vi "Cluster to String.vi"(1 "Correlator Initial Data":T1={"Max Exposition Time (ms)"=1, "Channel1 Threshold Voltage (mV)"=1, "Channel1 Pulse Front"="", "Channel2 Threshold Voltage (mV)"=1, "Channel2 Pulse Front"="", "Channel3 Threshold Voltage (mV)"=1, "Channel3 Pulse Front "="", "Channel4 Threshold Voltage (mV)"=1, "Channel4 Pulse Front "="", "Single Count Enable"={"Channel1"=FALSE, "Channel2"=FALSE, "Channel3"=FALSE, "Channel4"=FALSE}, "Single Count Max"=1, "Sum Count Enable"={"Channel1"=FALSE, "Channel2"=FALSE, "Channel3"=FALSE, "Channel4"=FALSE}, "Sum Count Max"=1, "Start-Stop1 Multyplex"={"Stop Channel"="", "Start Channel"=""}, "Stop Delay 1 (ns)"=1, "Window Length 1 (ns)"=4, "Window Offset 1 (ns) "=4, "Conditional Correlation 1"="", "Histogram Bin 1"="", "Histogram Start 1 (ns) "=4, "Start-Stop2 Multyplex "={"Stop Channel"="", "Start Channel"=""}, "Stop Delay 2 (ns)"=1, "Window Length 2 (ns) "=4, "Window Offset 2 (ns) "=4, "Conditional Correlation 2"="", "Histogram Bin 2"="", "Histogram Start 2 (ns)  "=4, "Start-Stop3 Multyplex"={"Stop Channel"="", "Start Channel"=""}, "Stop Delay 3 (ns)"=1, "Window Length 3 (ns) "=4, "Window Offset 3 (ns) "=4, "Conditional Correlation 3"="", "Histogram Bin 3"="", "Histogram Start 3 (ns) "=4, "Start-Stop4 Multyplex"={"Stop Channel"="", "Start Channel"=""}, "Stop Delay 4 (ns)"=1, "Window Length 4 (ns)  "=4, "Window Offset 4 (ns) "=4, "Conditional Correlation 4"="", "Histogram Bin 4"="", "Histogram Start 4 (ns)  "=4, "Coincidence Count Enable"={"Start-Stop1"=FALSE, "Start-Stop2"=FALSE, "Start-Stop3"=FALSE, "Start-Stop4"=FALSE}, "Coincidence Count Max"=1, "Coincidence Sum Enable 2"={"Start-Stop1"=FALSE, "Start-Stop2"=FALSE, "Start-Stop3"=FALSE, "Start-Stop4"=FALSE}, "Coincidence Sum Max"=1, "Output Channel Enable"={"Channel1"=FALSE, "Channel2"=FALSE, "Channel3"=FALSE, "Channel4"=FALSE}, "Output Channel Inversion"={"Channel1"=FALSE, "Channel2"=FALSE, "Channel3"=FALSE, "Channel4"=FALSE, "Output"=FALSE}} {"Coincidence Sum Max" min=1 max=16777215 step=1 format="%.7e"; "Coincidence Count Max" min=1 max=16777215 step=1 format="%.7e"; "Histogram Start 4 (ns)" min=0 max=120000 step=2; "Window Offset 4 (ns)" min=0 max=120000 step=2; "Window Length 4 (ns)" min=4 max=60000 step=4; "Stop Delay 4 (ns)" min=0 max=1008 step=16; "Histogram Start 3 (ns)" min=0 max=120000 step=2; "Window Offset 3 (ns)" min=0 max=120000 step=2; "Window Length 3 (ns)" min=4 max=60000 step=4; "Stop Delay 3 (ns)" min=0 max=1008 step=16; "Histogram Start 2 (ns)" min=0 max=120000 step=2; "Window Offset 2 (ns)" min=0 max=120000 step=2; "Window Length 2 (ns)" min=4 max=60000 step=4; "Stop Delay 2 (ns)" min=0 max=1008 step=16; "Histogram Start 1 (ns)" min=0 max=120000 step=2; "Window Offset 1 (ns)" min=0 max=120000 step=2; "Window Length 1 (ns)" min=4 max=60000 step=4; "Stop Delay 1 (ns)" min=0 max=1008 step=16; "Sum Count Max" min=1 max=16777215 step=1 format="%.7e"; "Single Count Max" min=1 max=16777215 step=1 format="%.7e"; "Channel4 Threshold Voltage (mV)" min=0 max=5000 step=10; "Channel3 Threshold Voltage (mV)" min=0 max=5000 step=10; "Channel2 Threshold Voltage (mV)" min=0 max=5000 step=10; "Channel1 Threshold Voltage (mV)" min=0 max=5000 step=10; "Max Exposition Time (ms)" min=1 max=3600000000 step=1 format="%.9e"}) -> (0 "string":string)   [LabVIEW 2012]
panel:
  out "Input":i64[](array[numeric])
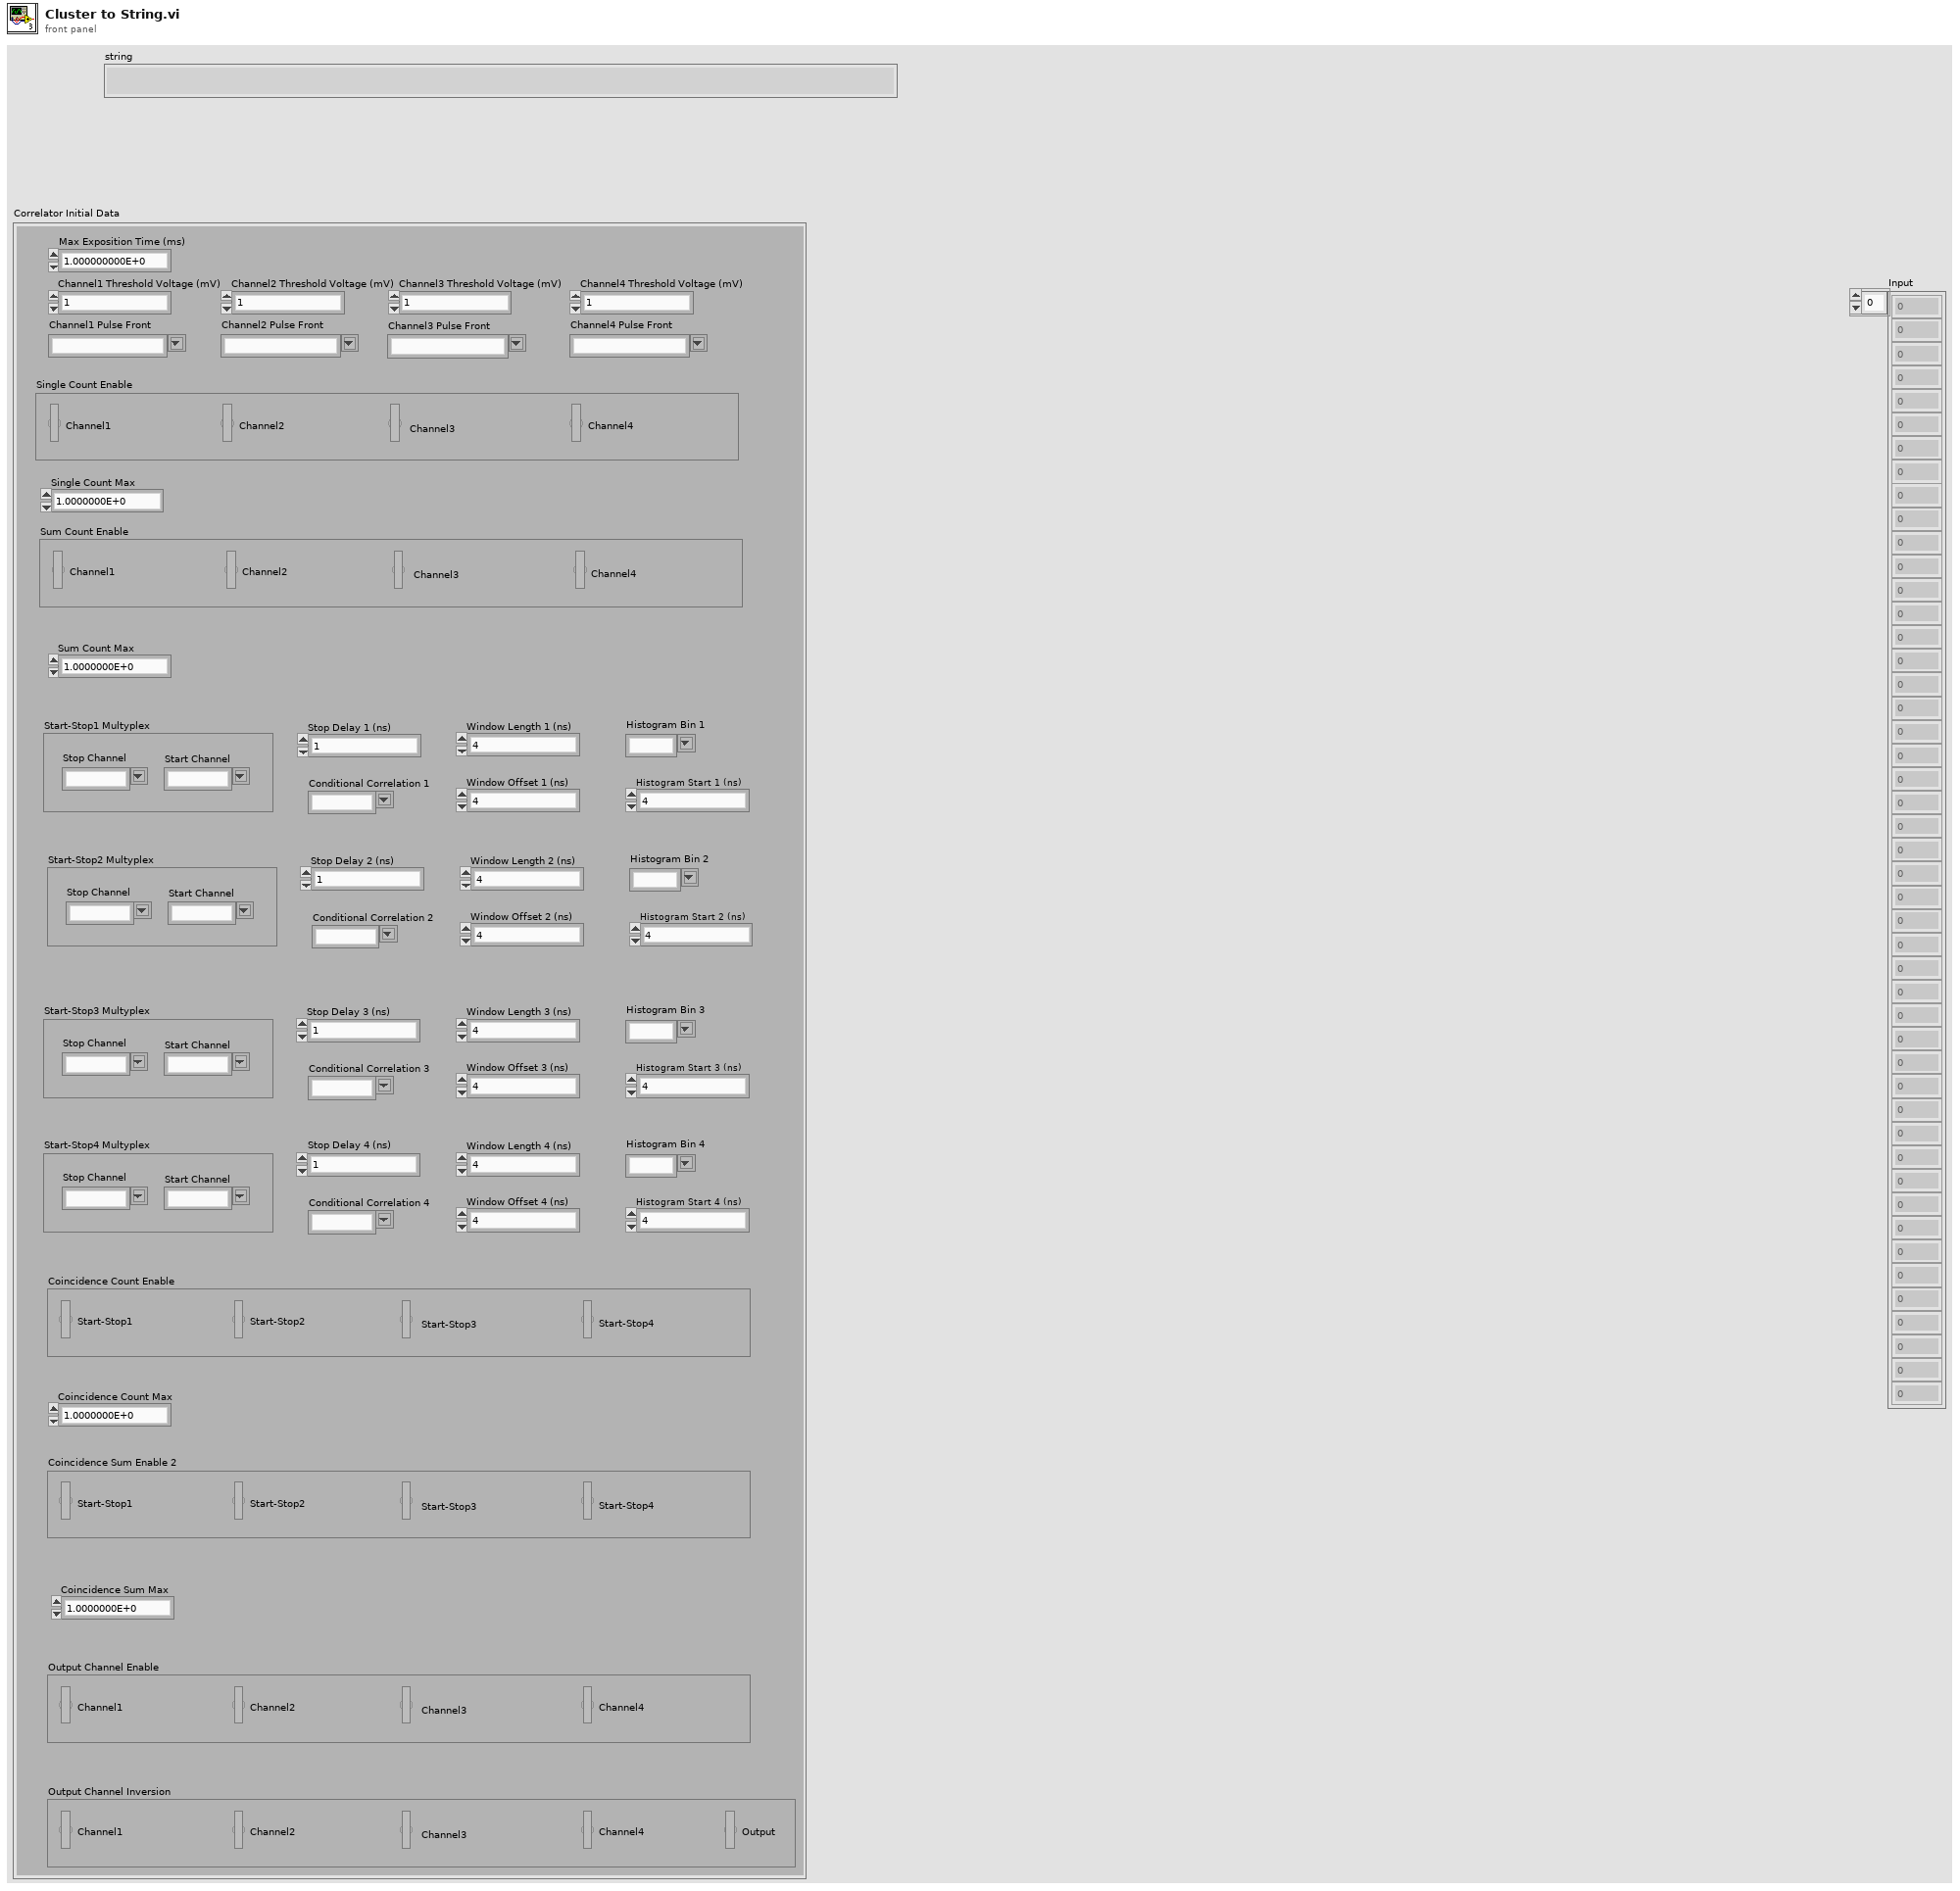
[diagram p1: front panel]
types:
  T1 = cluster{"Max Exposition Time (ms)":i64, "Channel1 Threshold Voltage (mV)":i32, "Channel1 Pulse Front":string, "Channel2 Threshold Voltage (mV)":i32, "Channel2 Pulse Front":string, "Channel3 Threshold Voltage (mV)":i32, "Channel3 Pulse Front ":string, "Channel4 Threshold Voltage (mV)":i32, "Channel4 Pulse Front ":string, "Single Count Enable":cluster{"Channel1":bool, "Channel2":bool, "Channel3":bool, "Channel4":bool}, "Single Count Max":i32, "Sum Count Enable":cluster{"Channel1":bool, "Channel2":bool, "Channel3":bool, "Channel4":bool}, "Sum Count Max":i32, "Start-Stop1 Multyplex":cluster{"Stop Channel":string, "Start Channel":string}, "Stop Delay 1 (ns)":i16, "Window Length 1 (ns)":i32, "Window Offset 1 (ns) ":i32, "Conditional Correlation 1":string, "Histogram Bin 1":string, "Histogram Start 1 (ns) ":i32, "Start-Stop2 Multyplex ":cluster{"Stop Channel":string, "Start Channel":string}, "Stop Delay 2 (ns)":i16, "Window Length 2 (ns) ":i32, "Window Offset 2 (ns) ":i32, "Conditional Correlation 2":string, "Histogram Bin 2":string, "Histogram Start 2 (ns)  ":i32, "Start-Stop3 Multyplex":cluster{"Stop Channel":string, "Start Channel":string}, "Stop Delay 3 (ns)":i16, "Window Length 3 (ns) ":i32, "Window Offset 3 (ns) ":i32, "Conditional Correlation 3":string, "Histogram Bin 3":string, "Histogram Start 3 (ns) ":i32, "Start-Stop4 Multyplex":cluster{"Stop Channel":string, "Start Channel":string}, "Stop Delay 4 (ns)":i16, "Window Length 4 (ns)  ":i32, "Window Offset 4 (ns) ":i32, "Conditional Correlation 4":string, "Histogram Bin 4":string, "Histogram Start 4 (ns)  ":i32, "Coincidence Count Enable":cluster{"Start-Stop1":bool, "Start-Stop2":bool, "Start-Stop3":bool, "Start-Stop4":bool}, "Coincidence Count Max":i32, "Coincidence Sum Enable 2":cluster{"Start-Stop1":bool, "Start-Stop2":bool, "Start-Stop3":bool, "Start-Stop4":bool}, "Coincidence Sum Max":i32, "Output Channel Enable":cluster{"Channel1":bool, "Channel2":bool, "Channel3":bool, "Channel4":bool}, "Output Channel Inversion":cluster{"Channel1":bool, "Channel2":bool, "Channel3":bool, "Channel4":bool, "Output":bool}}
  T2 = cluster{"Channel1":bool, "Channel2":bool, "Channel3":bool, "Channel4":bool}
  T3 = cluster{"Stop Channel":string, "Start Channel":string}
  T4 = cluster{"Start-Stop1":bool, "Start-Stop2":bool, "Start-Stop3":bool, "Start-Stop4":bool}
  T5 = cluster{"Channel1":bool, "Channel2":bool, "Channel3":bool, "Channel4":bool, "Output":bool}
  T6 = cluster{"Channel1 Pulse Front":string, "Channel2 Pulse Front":string, "Channel3 Pulse Front ":string, "Channel4 Pulse Front ":string, "Conditional Correlation 1":string, "Histogram Bin 1":string, "Conditional Correlation 2":string, "Histogram Bin 2":string, "Conditional Correlation 3":string, "Histogram Bin 3":string, "Conditional Correlation 4":string, "Histogram Bin 4":string}
  T7 = cluster{"Channel1 Pulse Front":u32, "Channel2 Pulse Front":u32, "Channel3 Pulse Front ":u32, "Channel4 Pulse Front ":u32, "Conditional Correlation 1":u32, "Histogram Bin 1":u32, "Conditional Correlation 2":u32, "Histogram Bin 2":u32, "Conditional Correlation 3":u32, "Histogram Bin 3":u32, "Conditional Correlation 4":u32, "Histogram Bin 4":u32}
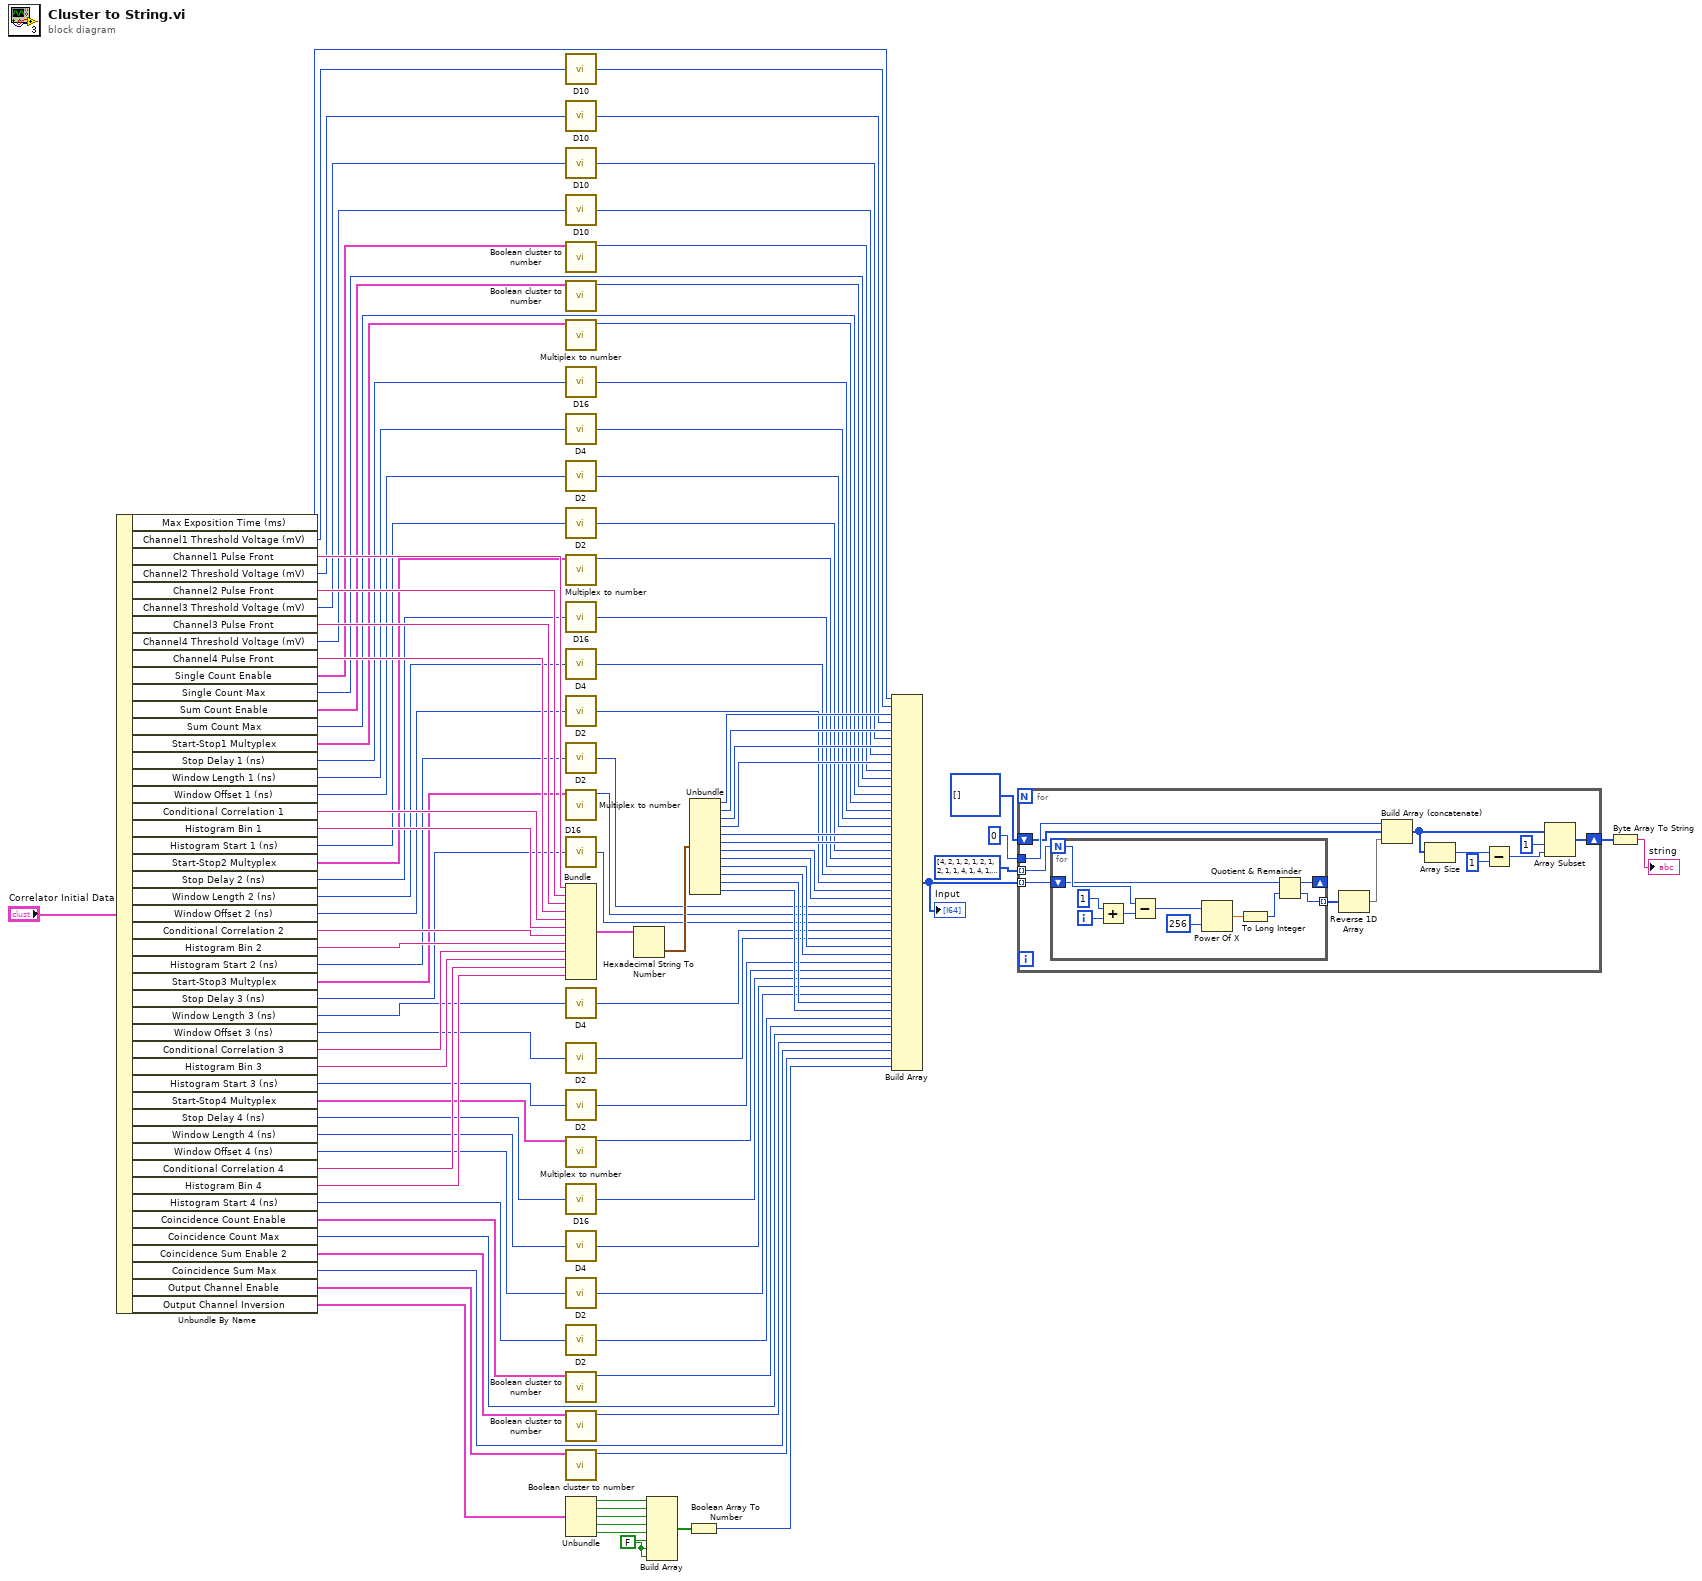
[diagram p0: block diagram]
diagram:
  w48 = FALSE ("element")
  n1 = Unbundle By Name("Correlator Initial Data") -> ("Max Exposition Time (ms)"=w76:i64, "Channel1 Threshold Voltage (mV)"=w75:i32, "Channel1 Pulse Front"=w105:string, "Channel2 Threshold Voltage (mV)"=w74:i32, "Channel2 Pulse Front"=w104:string, "Channel3 Threshold Voltage (mV)"=w73:i32, "Channel3 Pulse Front"=w103:string, "Channel4 Threshold Voltage (mV)"=w72:i32, "Channel4 Pulse Front"=w102:string, "Single Count Enable"=w42:T2, "Single Count Max"=w71:i32, "Sum Count Enable"=w41:T2, "Sum Count Max"=w70:i32, "Start-Stop1 Multyplex"=w81:T3, "Stop Delay 1 (ns)"=w69:i16, "Window Length 1 (ns)"=w68:i32, "Window Offset 1 (ns)"=w67:i32, "Conditional Correlation 1"=w101:string, "Histogram Bin 1"=w100:string, "Histogram Start 1 (ns)"=w66:i32, "Start-Stop2 Multyplex"=w79:T3, "Stop Delay 2 (ns)"=w65:i16, "Window Length 2 (ns)"=w64:i32, "Window Offset 2 (ns)"=w63:i32, "Conditional Correlation 2"=w99:string, "Histogram Bin 2"=w98:string, "Histogram Start 2 (ns)"=w62:i32, "Start-Stop3 Multyplex"=w77:T3, "Stop Delay 3 (ns)"=w61:i16, "Window Length 3 (ns)"=w60:i32, "Window Offset 3 (ns)"=w59:i32, "Conditional Correlation 3"=w97:string, "Histogram Bin 3"=w96:string, "Histogram Start 3 (ns)"=w58:i32, "Start-Stop4 Multyplex"=w82:T3, "Stop Delay 4 (ns)"=w57:i16, "Window Length 4 (ns)"=w56:i32, "Window Offset 4 (ns)"=w55:i32, "Conditional Correlation 4"=w95:string, "Histogram Bin 4"=w94:string, "Histogram Start 4 (ns)"=w54:i32, "Coincidence Count Enable"=w45:T4, "Coincidence Count Max"=w20:i32, "Coincidence Sum Enable 2"=w43:T4, "Coincidence Sum Max"=w22:i32, "Output Channel Enable"=w44:T2, "Output Channel Inversion"=w47:T5)
  n2 = call "D10.vi"("x"=w75) -> ("64bit integer"=w35:i64)
  n3 = call "D10.vi"("x"=w74) -> ("64bit integer"=w34:i64)
  n4 = call "D10.vi"("x"=w73) -> ("64bit integer"=w33:i64)
  n5 = call "D10.vi"("x"=w72) -> ("64bit integer"=w32:i64)
  n6 = call "Boolean cluster to number.vi"("Output Channel Enable"=w42) -> ("Numeric"=w84:u32)  [unwired: 10 in]
  n7 = call "Boolean cluster to number.vi"("Output Channel Enable"=w41) -> ("Numeric"=w83:u32)  [unwired: 10 in]
  n8 = call "Multiplex to number.vi"("Start-Stop4 Multyplex"=w81) -> ("Numeric"=w80:u32)  [unwired: 10 in]
  n9 = call "D16.vi"("x"=w69) -> ("64bit integer"=w31:i64)
  n10 = call "D4.vi"("x"=w68) -> ("64bit integer"=w30:i64)
  n11 = call "D2.vi"("x"=w67) -> ("64bit integer"=w29:i64)
  n12 = call "D2.vi"("x"=w66) -> ("64bit integer"=w28:i64)
  n13 = call "Multiplex to number.vi"("Start-Stop4 Multyplex"=w79) -> ("Numeric"=w78:u32)  [unwired: 10 in]
  n14 = call "D16.vi"("x"=w65) -> ("64bit integer"=w27:i64)
  n15 = call "D4.vi"("x"=w64) -> ("64bit integer"=w26:i64)
  n16 = call "D2.vi"("x"=w63) -> ("64bit integer"=w25:i64)
  n17 = call "D2.vi"("x"=w62) -> ("64bit integer"=w4:i64)
  n18 = call "Multiplex to number.vi"("Start-Stop4 Multyplex"=w77) -> ("Numeric"=w5:u32)  [unwired: 10 in]
  n19 = call "D16.vi"("x"=w61) -> ("64bit integer"=w6:i64)
  n20 = Bundle("Channel1 Pulse Front"=w105, "Channel2 Pulse Front"=w104, "Channel3 Pulse Front"=w103, "Channel4 Pulse Front"=w102, "Conditional Correlation 1"=w101, "Histogram Bin 1"=w100, "Conditional Correlation 2"=w99, "Histogram Bin 2"=w98, "Conditional Correlation 3"=w97, "Histogram Bin 3"=w96, "Conditional Correlation 4"=w95, "Histogram Bin 4"=w94) -> (w93:T6)  [unwired: 1 in]
  n21 = call "D4.vi"("x"=w60) -> ("64bit integer"=w7:i64)
  n22 = call "D2.vi"("x"=w59) -> ("64bit integer"=w8:i64)
  n23 = call "D2.vi"("x"=w58) -> ("64bit integer"=w11:i64)
  n24 = call "Multiplex to number.vi"("Start-Stop4 Multyplex"=w82) -> ("Numeric"=w12:u32)  [unwired: 10 in]
  n25 = call "D16.vi"("x"=w57) -> ("64bit integer"=w13:i64)
  n26 = call "D4.vi"("x"=w56) -> ("64bit integer"=w14:i64)
  n27 = call "D2.vi"("x"=w55) -> ("64bit integer"=w15:i64)
  n28 = call "D2.vi"("x"=w54) -> ("64bit integer"=w18:i64)
  n29 = call "Boolean cluster to number.vi"("Output Channel Enable"=w45) -> ("Numeric"=w19:u32)  [unwired: 10 in]
  n30 = call "Boolean cluster to number.vi"("Output Channel Enable"=w43) -> ("Numeric"=w21:u32)  [unwired: 10 in]
  n31 = call "Boolean cluster to number.vi"("Output Channel Enable"=w44) -> ("Numeric"=w23:u32)  [unwired: 10 in]
  n32 = Unbundle(w47) -> ("Channel1"=w50:bool, "Channel2"=w51:bool, "Channel3"=w52:bool, "Channel4"=w53:bool, "Output"=w46:bool)
  n33 = Hexadecimal String To Number(string=w93) -> (number=w92:T7)  [unwired: 2 in, 1 out]
  n34 = Build Array(w50, w51, w52, w53, w46, w48, w48, w48) -> (w49:bool[])
  n35 = Boolean Array To Number(Boolean array=w49) -> (number=w24:u32)
  n36 = Unbundle(w92) -> ("Channel1 Pulse Front"=w90:u32, "Channel2 Pulse Front"=w89:u32, "Channel3 Pulse Front"=w88:u32, "Channel4 Pulse Front"=w87:u32, "Conditional Correlation 1"=w86:u32, "Histogram Bin 1"=w85:u32, "Conditional Correlation 2"=w2:u32, "Histogram Bin 2"=w3:u32, "Conditional Correlation 3"=w9:u32, "Histogram Bin 3"=w10:u32, "Conditional Correlation 4"=w16:u32, "Histogram Bin 4"=w17:u32)
  n37 = Build Array(w76, w35, w90, w34, w89, w33, w88, w32, w87, w84, w71, w83, w70, w80, w31, w30, w29, w86, w85, w28, w78, w27, w26, w25, w2, w3, w4, w5, w6, w7, w8, w9, w10, w11, w12, w13, w14, w15, w16, w17, w18, w19, w20, w21, w22, w23, w24) -> (w1:i64[])
  "Input" <- w1
  n38 = for {
    tunnel: i8[] [4, 2, 1, 2, 1, 2, 1, 2, 1, 1, 4, 1, 4, 1, 1, 2, 2, 1, 1, 2, 1, 1, 2, 2, 1, 1, 2, 1, 1, 2, 2, 1, 1, 2, 1, 1, 2, 2, 1, 1, 2, 1, 4, 1, 4, 1, 1] ("Length array") -> [w117] mode=indexing
    tunnel: w1 -> [w116] mode=indexing
    shift-right: [w109] -> w38
    shift-left: i8[] [] -> [w114]
    tunnel: 0 -> [w115]
    n39 = for {
      N: w117 -> [w128]
      tunnel: [w118] -> w107 mode=indexing
      shift-right: [w121] -> _
      shift-left: w116 -> [w122]
      i -> [w127]
      n40 = Add(x=1, y=w127) -> (x+y=w125:i32)
      n41 = Subtract(x=w128, y=w125) -> (x-y=w124:i32)
      n42 = Power Of X(1:256 ("x"), 2:w124) -> (0:w120:dbl)
      n43 = To Long Integer(number=w120) -> (32bit integer=w119:i32)
      n44 = Quotient & Remainder(x=w122, y=w119) -> (x-y*floor(x/y)=w121:i64, floor(x/y)=w118:i64)
    }
    n45 = Reverse 1D Array(array=w107) -> (reversed array=w106:i64[])
    n46 = Build Array (concatenate)(w115, w114, w106) -> (w108:i64[])
    n47 = Array Size(array=w108) -> (size(s)=w112:i32)
    n48 = Subtract(x=w112, y=1) -> (x-y=w110:i32)
    n49 = Array Subset(array=w108, index=1, length=w110) -> (w109:i64[])
  }
  n50 = Byte Array To String(unsigned byte array=w38) -> (string=→"string":string)
